vi "PSPOP_Demo.vi"() -> ()   [LabVIEW 2016]
doc: "Demo for Type Sensitive Popup"
uses:
  Private/Ctrls/PSPOP_Grid.Cell Info.ctl
  Private/Ctrls/POP_Data Type.ctl
panel:
  out "数值":dbl
  in  "Popups":T1 {"Time" format="%<%Y/%m/%d %I:%M:%S>T"; "Boolean" items=["False", "True"]; "Ring" items=["Voltage", "Temperature", "Strain", "Current", "Resistance", "Frequency", "Position", "Acceleration", "Custom with Excitation", "Sound Pressure"]}
  in  "Cell Info (type only)":T2={"Tag"="", "Row"=0, "Column"=0, "In Symbol?"=FALSE, "In Data?"=FALSE, "Cell String"="", "Ctl Refnum"=refnum, "Prop Type"=enum."Unkown", "Ring Strings"=[], "Ring Values"=[], "New Cell String"=""}
  in  "stop":bool
  in  "Signal Settings":i32(listbox)=5
  # "Boolean Colors"
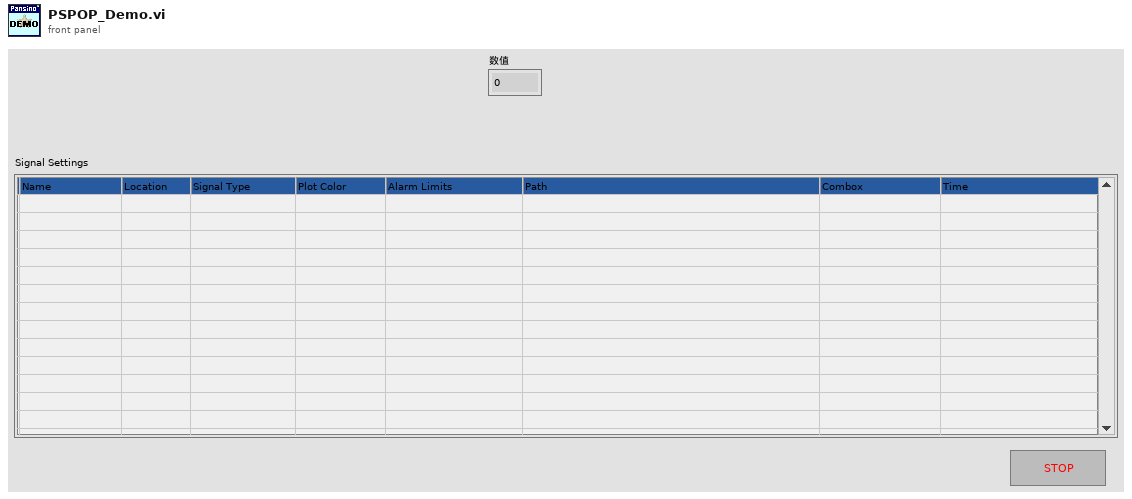
[diagram p1: front panel]
types:
  T1 = cluster{"Unknown":bool, "Unknown 2":bool, "String":string, "Integer":i32, "Float":dbl, "Color":u32, "Boolean":u32, "Ring":u32, "Captioned String":cluster{"String":string, "OK":bool, "Cancel":bool}, "Captioned Integer":cluster{"First":i32, "OK":bool, "Cancel":bool}, "Boolean Colors":cluster{"False":cluster{"FG":u32, "BG":u32}, "True":cluster{"FG":u32, "BG":u32}, "T  to  F":cluster{"FG":u32, "BG":u32}, "F  to  T":cluster{"FG":u32, "BG":u32}, "OK":bool, "Cancel":bool}, "2-Int Cluster":cluster{"First":i32, "Second":i32, "OK":bool, "Cancel":bool}, "4-Int Cluster":cluster{"First":i32, "Second":i32, "Third":i32, "Fourth":i32, "OK":bool, "Cancel":bool}, "6-Dbl Cluster":cluster{"First":dbl, "Second":dbl, "Third":dbl, "Fourth":dbl, "Fourth 2":dbl, "Third 2":dbl, "OK":bool, "Cancel":bool}, "Path":path, "Combox":string, "Time":timestamp, "ShortCut":string}
  T2 = typedef "PSPOP_Grid.Cell Info.ctl" = cluster{"Tag":string, "Row":i32, "Column":i32, "In Symbol?":bool, "In Data?":bool, "Cell String":string, "Ctl Refnum":refnum<vi>, "Prop Type":T3, "Ring Strings":string[], "Ring Values":ext[], "New Cell String":string}
  T3 = typedef "POP_Data Type.ctl" = enum16{"NO POPUP", "Unkown", "String", "Integer", "Float", "Color", "Boolean", "Ring", "Captioned String", "Captioned Integer", "Button Color", "2 Int Cluster", "4 Int Cluster", "6-Dbl Cluster", "Path", "Combox", "Time", "ShotCut String"}
  T4 = typedef "LVPoint32TypeDef.ctl" = cluster{"Horizontal":i32, "Vertical":i32}
  T5 = typedef "POP_Popup Call Parameters.ctl" = cluster{"Prop Type":T3, "Initial Value":variant, "Caption Strings":string[], "Ring Strings":string[], "Cell Rect":cluster{"left":i16, "top":i16, "right":i16, "bottom":i16}, "Mouse Coords":cluster{"x":i16, "y":i16}, "Call Data":variant, "Ring Values":ext[], "Browse Options":T6, "Combo Box":cluster{"Allow Undefined Strings":bool}}
  T6 = typedef "LVBrowseOptionsTypeDef.ctl" = cluster{"Prompt":string, "Match Pattern":string, "Mode":enum32{"existing file", "new file", "new or existing file", "existing dir", "new dir", "new or existing dir", "existing file (use LLBs)", "new file (use LLBs)", "new or existing file (use LLBs)", "new or existing file or directory (use LLBs)", "existing dir (use LLBs)", "new dir (use LLBs)", "new or existing dir (use LLBs)", "existing file or dir", "new file or dir", "new or existing file or dir", "existing file or dir (use LLBs)", "new file or dir (use LLBs)"}, "Start Path":path, "Pattern Label":string, "Button Text":string}
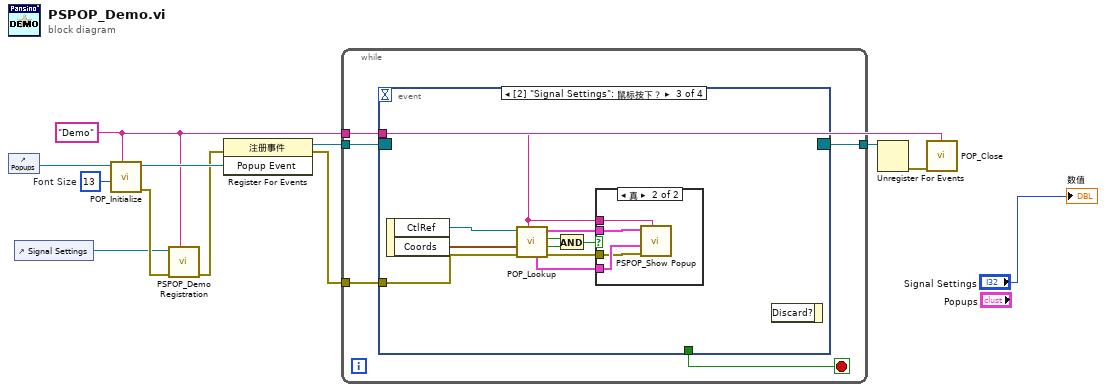
[diagram p0: block diagram]
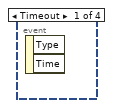
[diagram p2: hidden frame]
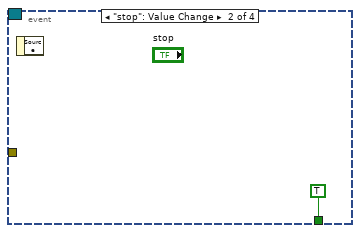
[diagram p3: hidden frame]
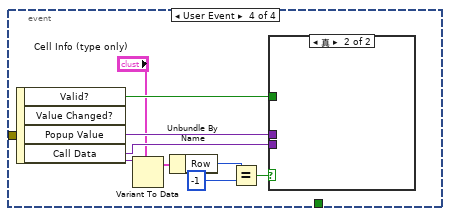
[diagram p5: hidden frame]
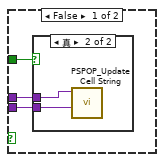
[diagram p6: hidden frame]
diagram:
  w3 = "Demo" ("Name")
  w11 = u32 13  # Font Size
  n1 = control-ref of="Popups"() -> (w12:refnum<vi>)
  n2 = control-ref of="Signal Settings"() -> (w2:refnum<vi>)
  n3 = call "POP_Initialize.vi"("Name"=w3, "Font Size"=w11, "Popup Cluster Ref"=w12) -> ("error out"=w6:errorcluster, "Popup Event"=w10:refnum<user-event>)  [unwired: 7 in]
  n4 = call "PSPOP_Demo Registration.vi"("Name"=w3, "error in (no error)"=w6, "Signal Settings ref"=w2) -> ("error out"=w5:errorcluster)  [unwired: 8 in]
  n5 = register-events(error in=w5, w10) -> (reference out=w9:refnum<event-registration>, error out=w4:errorcluster)  [unwired: 1 in]
  n6 = while {
    tunnel: w9 -> [w17]
    tunnel: [w16] -> w8
    tunnel: w4 -> [w13]
    tunnel: w3 -> [w14]
    stop <- w15 stop-if-true
    n7 = event shown="[2] \"Signal Settings\": 鼠标按下？" {
      selector: w17 -> [_ _ _ _]
      dyn-events: [_ _ _ _] -> w16
      timeout: _ -> [_ _ _ _]
      tunnel: [_ TRUE _ _] -> w15
      tunnel: w14 -> [_ _ w20 _]
      tunnel: w13 -> [_ _ w19 _]
      event Timeout {
        n8 = event-data() -> ()  [unwired: 1 in, 2 out]
      }
      event "stop": Value Change {
        n9 = event-data() -> ()  [unwired: 1 in, 1 out]
      }
      event "Signal Settings": Mouse Down? {
        n10 = event-data() -> ("CtlRef"=w28:refnum<vi>, "Coords"=w27:T4)  [unwired: 1 in]
        n11 = call "POP_Lookup.vi"("Name"=w20, "error in (no error)"=w19, "Point"=w27, "Ctl Refnum"=w28) -> ("error out"=w21:errorcluster, "In Bounds?"=w25:bool, "Found"=w26:bool, "Popup Parameters"=w23:T5, "Cell Info (Call data)"=w22:T2)  [unwired: 3 in]
        n12 = And(x=w26, y=w25) -> (x .and. y?=w24:bool)
        n13 = case shown="真" w24 {
          tunnel: w23 -> [_ w32]
          tunnel: w22 -> [_ w31]
          tunnel: w21 -> [_ w30]
          tunnel: w20 -> [_ w29]
          frame False {
          }
          frame True {
            n14 = call "PSPOP_Show Popup.vi"("Name"=w29, "error in (no error)"=w30, "Call Data (ignore if empty)"=w31, "Popup Parameters"=w32) -> ()  [unwired: 7 in, 1 out]
          }
        }
        n15 = event-data() -> ()  [unwired: 2 in, 1 out]
      }
      event User Event {
        n16 = event-data() -> ("Valid?"=w40:bool, "Popup Value"=w39:variant, "Call Data"=w38:variant)  [unwired: 1 in, 1 out]
        n17 = Variant To Data(type="Cell Info (type only)", Variant=w38) -> (data=w37:T2)  [unwired: 1 in, 1 out]
        n18 = Unbundle By Name(w37) -> ("Row"=w36:i32)
        n19 = Equal?(x=w36, y=-1) -> (x = y?=w34:bool)
        n20 = case shown="真" w34 {
          tunnel: w40 -> [w43 _]
          tunnel: w39 -> [w42 _]
          tunnel: w38 -> [w41 _]
          frame False {
            n21 = case shown="真" w43 {
              tunnel: w42 -> [_ w44]
              tunnel: w41 -> [_ w45]
              frame False {
              }
              frame True {
                n22 = call "PSPOP_Update Cell String.vi"("Call Data (must be Cell Info cluster)"=w45, "Popup Value"=w44) -> ()  [unwired: 8 in, 2 out]
              }
            }
          }
          frame True {
          }
        }
      }
    }
  }
  n23 = Unregister For Events(event registration refnum=w8) -> (error out=w7:errorcluster)  [unwired: 1 in]
  n24 = call "POP_Close.vi"("Name"=w3, "error in (no error)"=w7) -> ()  [unwired: 9 in, 1 out]
  "数值" <- "Signal Settings"
